vi "bats.orderbook.vi"(10 "data_valid":bool, 11 "data":u8) -> (1 "tlast":bool, 2 "tvalid":bool, 3 "tdata":u8)   [LabVIEW 2020]
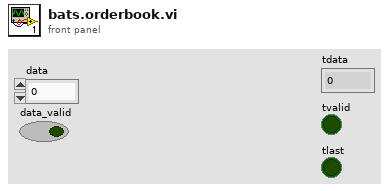
[diagram p1: front panel]
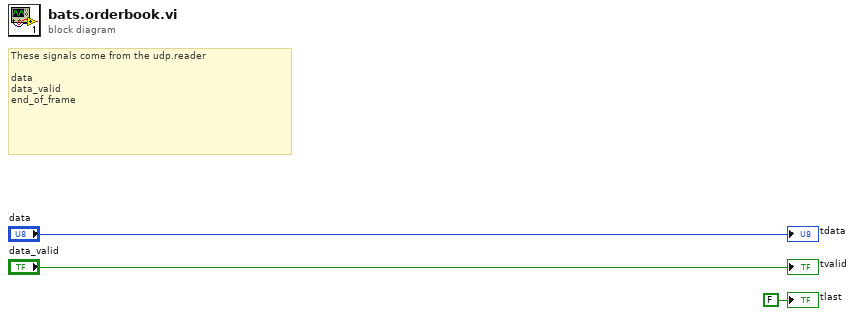
[diagram p0: block diagram]
diagram:
  # "These signals come from the udp.reader\n\ndata\ndata_valid\nend_of_frame"
  "tdata" <- "data"
  "tvalid" <- "data_valid"
  "tlast" <- FALSE ("tlast")
